vi "create_file_name (SubVI).vi"(4 "Use electrode config?":bool, 6 "file_idx":i32, 8 "num files":i32, 9 "base name":string, 10 "Path":path, 11 "Cluster":T1) -> (3 "out path":path)   [LabVIEW 2014]
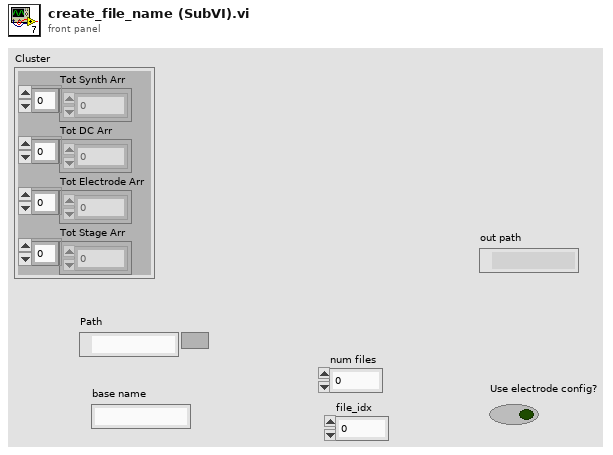
[diagram p1: front panel]
types:
  T1 = cluster{"Tot Synth Arr":dbl[], "Tot DC Arr":dbl[], "Tot Electrode Arr":dbl[], "Tot Stage Arr":dbl[]}
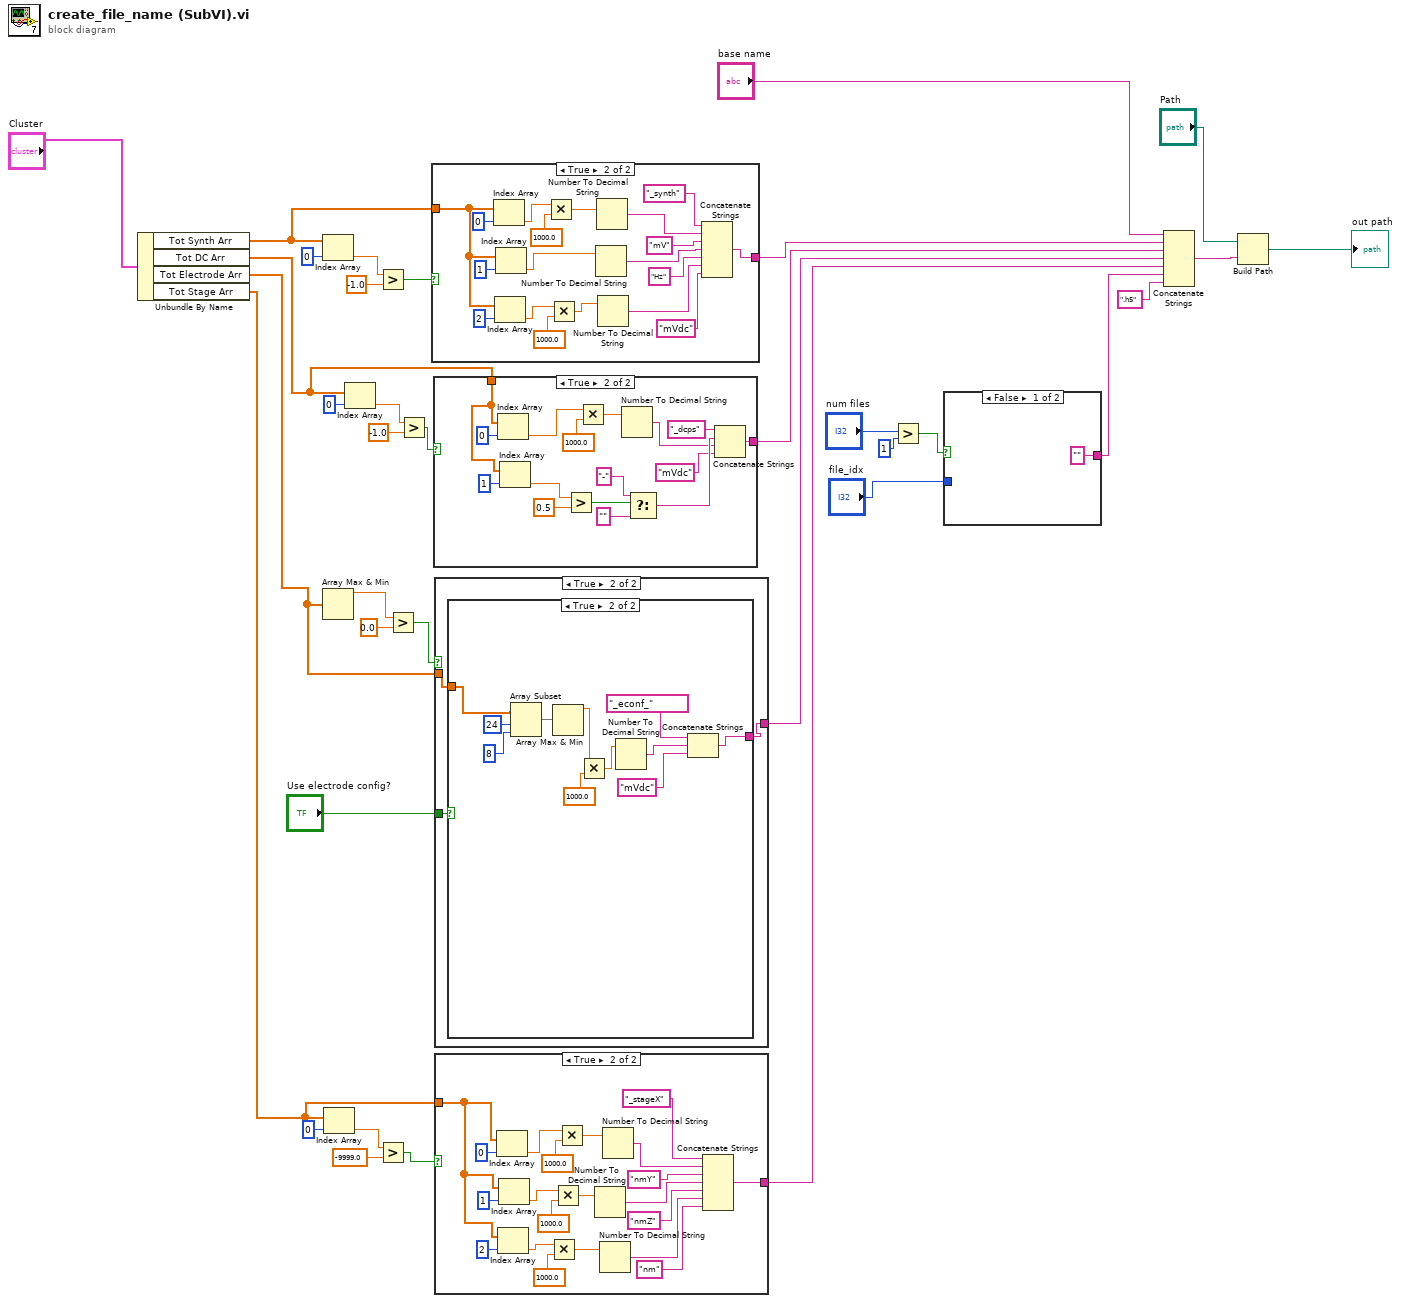
[diagram p0: block diagram]
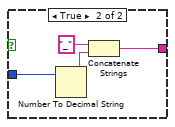
[diagram p2: hidden frame]
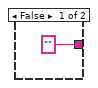
[diagram p3: hidden frame]
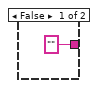
[diagram p4: hidden frame]
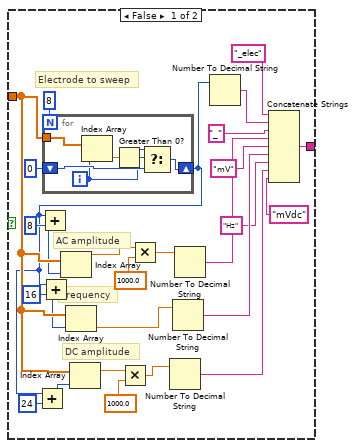
[diagram p5: hidden frame]
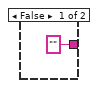
[diagram p6: hidden frame]
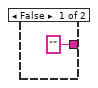
[diagram p7: hidden frame]
diagram:
  n1 = Unbundle By Name("Cluster") -> ("Tot Synth Arr"=w30:dbl[], "Tot DC Arr"=w25:dbl[], "Tot Electrode Arr"=w3:dbl[], "Tot Stage Arr"=w18:dbl[])
  n2 = Index Array(array=w30, index=0) -> (element=w32:dbl)
  n3 = Array Max & Min(array=w3) -> (max value=w2:dbl)  [unwired: 3 out]
  n4 = Index Array(array=w18, index=0) -> (element=w20:dbl)
  n5 = Index Array(array=w25, index=0) -> (element=w27:dbl)
  n6 = Greater?(x=w32, y=-1.0) -> (0:w31:bool)
  n7 = Greater?(x=w20, y=-9999.0) -> (0:w19:bool)
  n8 = Greater?(x=w2, y=0.0) -> (0:w23:bool)
  n9 = Greater?(x=w27, y=-1.0) -> (0:w26:bool)
  n10 = case shown="True" w31 {
    tunnel: w30 -> [_ w55]
    tunnel: ["" w37] -> w16
    frame False {
    }
    frame True {
      n11 = Index Array(array=w55, index=0) -> (element=w50:dbl)
      n12 = Index Array(array=w55, index=2) -> (element=w46:dbl)
      n13 = Index Array(array=w55, index=1) -> (element=w51:dbl)
      n14 = Multiply(x=w50, y=1000.0) -> (x*y=w49:dbl)
      n15 = Multiply(x=w46, y=1000.0) -> (x*y=w45:dbl)
      n16 = Number To Decimal String(number=w51) -> (decimal integer string=w41:string)  [unwired: 1 in]
      n17 = Number To Decimal String(number=w49) -> (decimal integer string=w43:string)  [unwired: 1 in]
      n18 = Number To Decimal String(number=w45) -> (decimal integer string=w39:string)  [unwired: 1 in]
      n19 = Concatenate Strings("_synth" ("string"), w43, "mV" ("string"), w41, "Hz" ("string"), w39, "mVdc" ("string")) -> (w37:string)
    }
  }
  n20 = case shown="True" w26 {
    tunnel: w25 -> [_ w70]
    tunnel: ["" w57] -> w15
    frame False {
    }
    frame True {
      n21 = Index Array(array=w70, index=0) -> (element=w68:dbl)
      n22 = Index Array(array=w70, index=1) -> (element=w64:dbl)
      n23 = Greater?(x=w64, y=0.5) -> (0:w63:bool)
      n24 = Multiply(x=w68, y=1000.0) -> (x*y=w67:dbl)
      n25 = Number To Decimal String(number=w67) -> (decimal integer string=w59:string)  [unwired: 1 in]
      n26 = Select(t="-" ("string"), s=w63, f="" ("string")) -> (s? t:f=w60:string)
      n27 = Concatenate Strings("_dcps" ("string"), w60, w59, "mVdc" ("string")) -> (w57:string)
    }
  }
  n28 = case shown="True" w23 {
    tunnel: w3 -> [_ w76]
    tunnel: ["" w75] -> w14
    tunnel: "Use electrode config?" -> [_ w74]
    frame False {
    }
    frame True {
      n29 = case shown="True" w74 {
        tunnel: w76 -> [w103 w118]
        tunnel: [w86 w119] -> w75
        frame False {
          # "DC amplitude"
          # "Frequency"
          # "AC amplitude"
          # "Electrode to sweep"
          n30 = for {
            N: 8 -> [_]
            tunnel: w103 -> [w109]
            shift-right: [w105] -> w78
            shift-left: 0 -> [w106]
            i -> [w104]
            n31 = Index Array(array=w109, index=w104) -> (element=w108:dbl)
            n32 = Greater Than 0?(x=w108) -> (x > 0?=w107:bool)
            n33 = Select(t=w104, s=w107, f=w106) -> (s? t:f=w105:i32)
          }
          n34 = Add(x=w78, y=24) -> (x+y=w79:i32)
          n35 = Add(x=w78, y=8) -> (x+y=w83:i32)
          n36 = Add(x=w78, y=16) -> (x+y=w81:i32)
          n37 = Index Array(array=w103, index=w83) -> (element=w97:dbl)
          n38 = Index Array(array=w103, index=w81) -> (element=w95:dbl)
          n39 = Index Array(array=w103, index=w79) -> (element=w94:dbl)
          n40 = Multiply(x=w94, y=1000.0) -> (x*y=w93:dbl)
          n41 = Multiply(x=w97, y=1000.0) -> (x*y=w96:dbl)
          n42 = Number To Decimal String(number=w93) -> (decimal integer string=w88:string)  [unwired: 1 in]
          n43 = Number To Decimal String(number=w95) -> (decimal integer string=w90:string)  [unwired: 1 in]
          n44 = Number To Decimal String(number=w96) -> (decimal integer string=w92:string)  [unwired: 1 in]
          n45 = Number To Decimal String(number=w78) -> (decimal integer string=w101:string)  [unwired: 1 in]
          n46 = Concatenate Strings("_elec" ("string"), w101, "_" ("string"), w92, "mV" ("string"), w90, "Hz" ("string"), w88, "mVdc" ("string")) -> (w86:string)
        }
        frame True {
          n47 = Array Subset(array=w118, index=24, length=8) -> (w115:dbl[])
          n48 = Array Max & Min(array=w115) -> (max value=w113:dbl)  [unwired: 3 out]
          n49 = Multiply(x=w113, y=1000.0) -> (x*y=w112:dbl)
          n50 = Number To Decimal String(number=w112) -> (decimal integer string=w111:string)  [unwired: 1 in]
          n51 = Concatenate Strings("_econf_", w111, "mVdc" ("string")) -> (w119:string)
        }
      }
    }
  }
  n52 = case shown="True" w19 {
    tunnel: w18 -> [_ w139]
    tunnel: ["" w122] -> w13
    frame False {
    }
    frame True {
      n53 = Index Array(array=w139, index=0) -> (element=w137:dbl)
      n54 = Index Array(array=w139, index=2) -> (element=w134:dbl)
      n55 = Index Array(array=w139, index=1) -> (element=w133:dbl)
      n56 = Multiply(x=w134, y=1000.0) -> (x*y=w130:dbl)
      n57 = Multiply(x=w133, y=1000.0) -> (x*y=w131:dbl)
      n58 = Multiply(x=w137, y=1000.0) -> (x*y=w132:dbl)
      n59 = Number To Decimal String(number=w131) -> (decimal integer string=w126:string)  [unwired: 1 in]
      n60 = Number To Decimal String(number=w130) -> (decimal integer string=w124:string)  [unwired: 1 in]
      n61 = Number To Decimal String(number=w132) -> (decimal integer string=w128:string)  [unwired: 1 in]
      n62 = Concatenate Strings("_stageX", w128, "nmY" ("string"), w126, "nmZ" ("string"), w124, "nm" ("string")) -> (w122:string)
    }
  }
  n63 = Greater?(x="num files", y=1) -> (0:w7:bool)
  n64 = case shown="False" w7 {
    tunnel: "file_idx" -> [_ w146]
    tunnel: ["" w144] -> w5
    frame False {
    }
    frame True {
      n65 = Number To Decimal String(number=w146) -> (decimal integer string=w145:string)  [unwired: 1 in]
      n66 = Concatenate Strings("_" ("string"), w145) -> (w144:string)
    }
  }
  n67 = Concatenate Strings("base name", w16, w15, w14, w13, w5, ".h5" ("string")) -> (w12:string)
  n68 = Build Path(base path="Path", name or relative path=w12) -> (appended path=→"out path":path)
